vi "STAGE+mono+counter_edit20.vi"() -> ()   [LabVIEW 2017]
panel:
  out "PROGRESS":u8(slide) max=10 step=10 scale=0.0..100.0
  in  "?":enum32{"Page 1", "Page 2"}(tab)
  out "XY Graph":cluster{dbl[], dbl[]}(graph)
  out "XY Graph 2":cluster{dbl[], dbl[]}[](graph)
  in  "Collect Data!":bool
  out "Timeout":bool
  in  "?":bool
  out "Timeout 2":bool
  out "Waveform Graph":waveform(dbl)[](graph)
  in  "?":enum32{"DELAY", "COUNTER", "MONO", "PLOT"}(tab)
  out "Final time [ps]":dbl
  out "Current time [ps]":dbl
  out "Initial time [ps]":dbl
  in  "Set this as t0":bool
  in  "Axis":i32=1
  in  "Motor ON":bool
  in  "Motor OFF":bool
  out "Current Position [mm]":dbl
  out "Final Position [mm]":dbl
  in  "Data Points":i32=100
  out "Current Point":i32
  in  "Step Size [um]":i32=10
  in  "Target [mm]":dbl format="%.3f"
  in  "Move":bool
  out "Initial position [mm]":dbl
  in  "GPIB address":string="23"
  in  "Count Mode":u16(ring) items=["A,B for Preset T", "A-B for Preset T", "A+B for Preset T", "A for Preset B"]
  in  "Trigger mode":u16(ring) items=["10 MHz"=0, "Input 2"=2, "Input T"=3]
  in  "Channel A Input":u16(ring)=1 items=["10 MHz", "Input 1"]
  in  "Channel B Input":u16(ring)=2 items=["Input 1"=1, "Input 2"=2]
  in  "Number of Measurements\n to take at one point/ Number of Periods":u16=1 min=1 max=2000 step=1
  in  "Time between measurements\n at one point (s)/Dwell Time":dbl=0.002 min=0.002 max=60.0 step=0.001
  in  "gate mode (CW:0)":i16(slide) scale=0.0..2.0 scale format="%.2f"
  out "Counts":i32
  in  "Integrating time \nin 10^-7 sec":dbl=10000000.0
  in  "Discriminator Level (mV)":dbl min=-300.0 max=300.0 step=0.2
  in  "Discriminator Slope":bool
  in  "Channel":i16 min=0 max=2 step=1
  out "Grating #":dbl
  out "Blaze angle":dbl
  out "Grooves/mm":dbl
  out "Mono port":T1(ring)
  out "Time delay":u32=450000 min=1
  in  "Step size":dbl=10.0 min=0.0
  in  "Scan to":i32=4000
  in  "Scan from":i32=2600
  out "Current wavelength":dbl
  in  "?":bool
  in  "Array":dbl[](array[numeric])
  out "Numeric":i32
  out "Numeric 2":i32
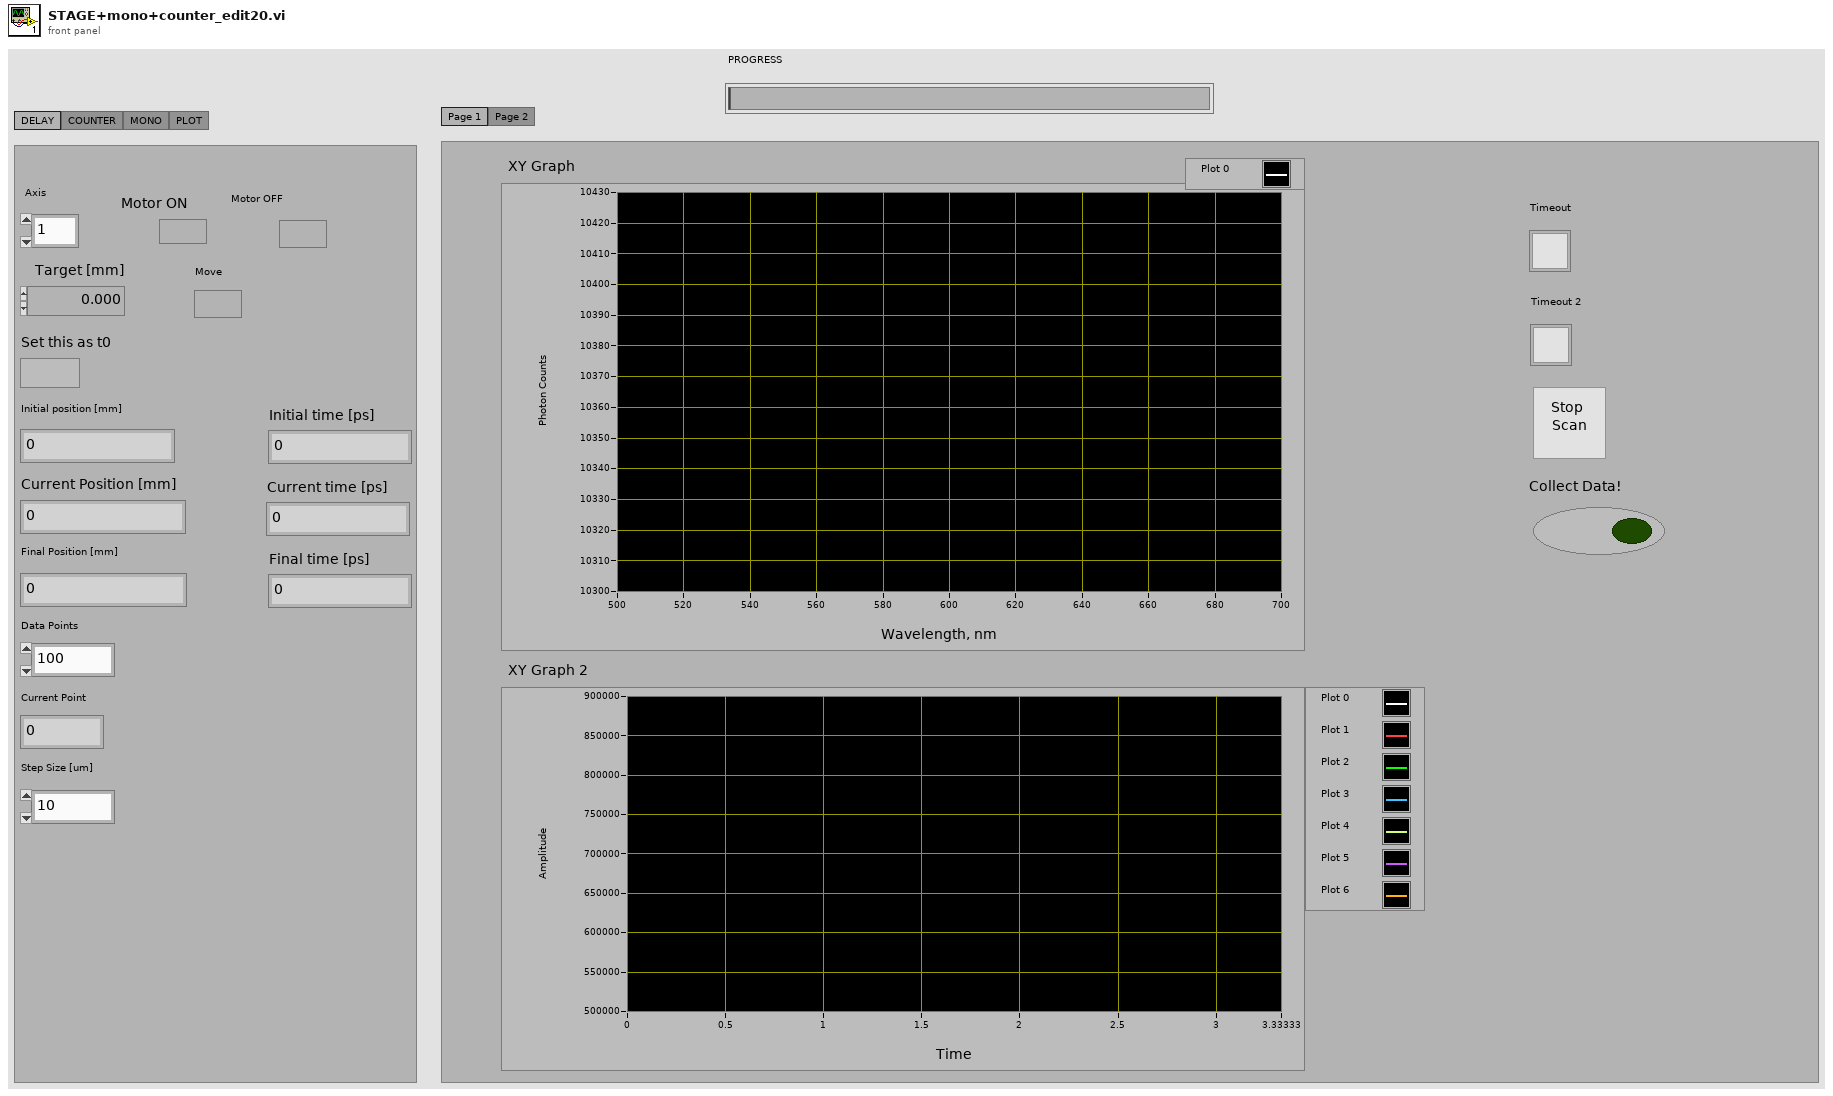
[diagram p1: front panel]
types:
  T1 = enum8{"COM 1", "COM 2", "COM 3", "COM 4", "COM 5", "COM 6", "COM 7", "COM 8", "COM 9"}
  T2 = cluster{"input XON/XOFF":bool, "input HW Handshake":bool, "input alt HW HShk":bool, "output XON/XOFF":bool, "output HW Handshake":bool, "output alt HW HShk":bool, "XOFF byte":u8, "XON byte":u8, "parity error byte":u16}
  T3 = enum16{"no parity", "odd parity", "even parity", "mark parity", "space parity"}
  T4 = typedef "NI_Matrix.lvlib/RealMatrix.ctl" = dbl[][]
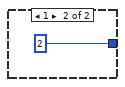
[diagram p5: hidden frame]
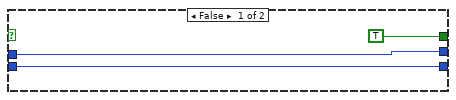
[diagram p6: hidden frame]
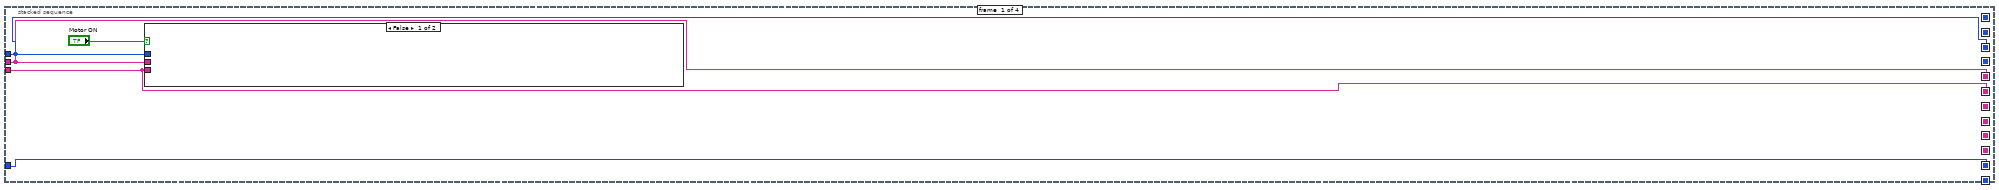
[diagram p7: hidden frame]
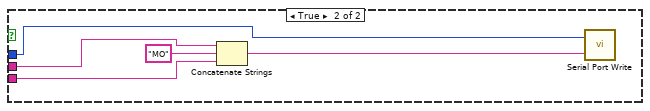
[diagram p8: hidden frame]
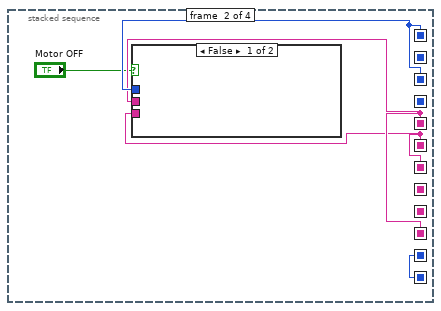
[diagram p9: hidden frame]
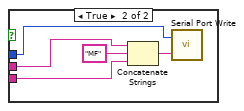
[diagram p10: hidden frame]
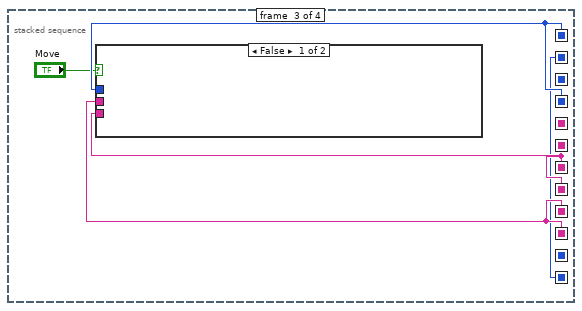
[diagram p11: hidden frame]
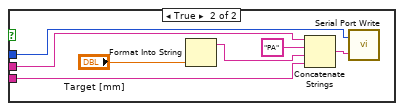
[diagram p12: hidden frame]
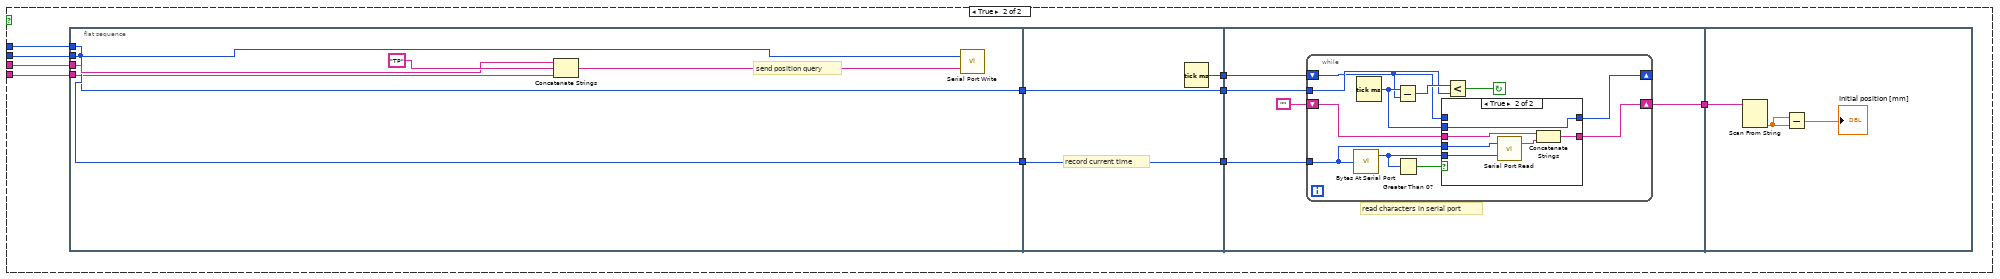
[diagram p13: hidden frame]
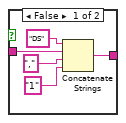
[diagram p15: hidden frame]
diagram:
  (unwired) FALSE
  w41 = u32 19200  # baud rate
  w40 = u16 8  # data bits
  w39 = enum16{"1 bit", "1.5 bits", "2 bits"}."1 bit"  # stop bits
  w43 = T3."no parity"  # parity
  w38 = 4  # 0=COM1 so n=COM(n+1)
  w42 = u16 1024  # buffer size
  n1 = flat-sequence {
    tunnel: ["Data Points"] -> w47
    tunnel: "Axis" -> [w69]
    tunnel: [w61] -> w46
    tunnel: [w69] -> w45
    tunnel: ["Step Size [um]"] -> w19
    tunnel: [w61] -> w18
    tunnel: ["Step Size [um]"] -> w17
    tunnel: ["Data Points"] -> w16
    tunnel: [w61] -> w15
    tunnel: [w60] -> w14
    tunnel: [w61] -> w12
    tunnel: [w60] -> w11
    tunnel: [w63] -> w10
    tunnel: [w52] -> w9
    tunnel: [w53] -> w2
    tunnel: [w52] -> w1
    tunnel: w47 -> [w161]
    tunnel: w46 -> [w160]
    tunnel: w45 -> [w159]
    tunnel: w38 -> [w155]
    tunnel: "GPIB address" -> [w154]
    tunnel: "GPIB address" -> [w153]
    tunnel: w19 -> [w142]
    tunnel: w18 -> [w140]
    tunnel: w17 -> [w139]
    tunnel: w16 -> [w137]
    tunnel: w15 -> [w132]
    tunnel: w14 -> [w131]
    tunnel: "Integrating time \nin 10^-7 sec" -> [w130]
    tunnel: w12 -> [w129]
    tunnel: w11 -> [w128]
    tunnel: w10 -> [w127]
    tunnel: w9 -> [w125]
    tunnel: w5 -> [w115]
    tunnel: w4 -> [w114]
    tunnel: w3 -> [w113]
    tunnel: w2 -> [w83]
    tunnel: w1 -> [w82]
    frame #0 {
      n2 = while {
        stop <- "Collect Data!" stop-if-true
        n3 = Multiply(x=1, y=1000) -> (x*y=w51:i32)
        n4 = Wait (ms)(milliseconds to wait=w51) -> ()  [unwired: 1 out]
      }
    }
    frame #1 {
      w54 = 1000000000000.0
      w59 = 1000
      w62 = 300000000
      w64 = 1000
      n5 = local read "Initial position [mm]"() -> (w61:dbl)
      n6 = Multiply(x="Step Size [um]", y="Data Points") -> (x*y=w68:i32)
      n7 = Divide(x=w68, y=w64) -> (x/y=w67:dbl)
      n8 = Divide(x="Step Size [um]", y=w64) -> (x/y=w63:dbl)
      n9 = Add(x=w61, y=w67) -> (x+y=w60:dbl)
      "Final Position [mm]" <- w60
      n10 = Divide(x=w60, y=w59) -> (x/y=w58:dbl)
      n11 = Divide(x=w61, y=w59) -> (x/y=w57:dbl)
      n12 = Divide(x=w58, y=w62) -> (x/y=w55:dbl)
      n13 = Divide(x=w57, y=w62) -> (x/y=w56:dbl)
      n14 = Multiply(x=w55, y=w54) -> (x*y=w53:dbl)
      "Final time [ps]" <- w53
      n15 = Multiply(x=w56, y=w54) -> (x*y=w52:dbl)
      "Initial time [ps]" <- w52
    }
    frame #2 {
      w74 = 1
      w95 = "\r\n"
      n16 = Increment(x=w137) -> (x+1=w138:i32)
      n17 = local read "Numeric 2"() -> (w78:i32)
      n18 = Multiply(x="Scan from", y=w74) -> (x*y=w70:i32)
      n19 = Multiply(x="Scan to", y=w74) -> (x*y=w72:i32)
      n20 = local read "Numeric"() -> (w77:i32)
      n21 = Divide(x=w142, y=1000.0) -> (x/y=w119:dbl)
      n22 = for {
        N: w138 -> [_]
        tunnel: w119 -> [w172]
        tunnel: w140 -> [w170]
        tunnel: [w163] -> w136 mode=indexing
        i -> [w171]
        # "distances"
        n23 = Multiply(x=w172, y=w171) -> (x*y=w169:dbl)
        n24 = Add(x=w170, y=w169) -> (x+y=w168:dbl)
        n25 = Divide(x=w168, y=1000) -> (x/y=w162:dbl)
        n26 = Divide(x=w162, y=300000000) -> (x/y=w165:dbl)
        n27 = Multiply(x=w165, y=1000000000000.0) -> (x*y=w163:dbl)
      }
      n28 = To Time Stamp(1:w70) -> (0:w86:timestamp)
      n29 = Initialize Array(0.0, w77, w78) -> ()  [unwired: 1 out]
      n30 = Multiply(x=w72, y=1) -> (x*y=w126:i32)
      n31 = Multiply(x=1, y=w70) -> (x*y=w118:i32)
      n32 = Divide(x=w119, y=1000.0) -> (x/y=w120:dbl)
      n33 = Subtract(x=w126, y=w118) -> (x-y=w148:i32)
      n34 = Divide(x=w120, y=300000000) -> (x/y=w122:dbl)
      n35 = Divide(x=w148, y="Step size") -> (x/y=w147:dbl)
      n36 = Bundle By Name("Y"=dbl[] [], "t0"=w86, "dt"="Step size") -> (w85:waveform(dbl))  [unwired: 1 in]
      n37 = property on="Waveform Graph" class="WFGraph (strict)"("XScale.Increment"="Step size", "XScale.Maximum"=w72, "XScale.Minimum"=w70) -> ()  [unwired: 2 in, 2 out]
      n38 = Multiply(x=w122, y=1000000000000.0) -> (x*y=w81:dbl)
      n39 = Build Array(w85) -> (w84:waveform(dbl)[])
      n40 = Round Toward -Infinity(1:w147) -> (0:w146:dbl)
      n41 = Concatenate Strings("\r", "\n") -> (w156:string)
      n42 = property on="XY Graph 2" class="XYGraph (strict)"("XScale.Increment"=w81, "XScale.Maximum"=w83, "XScale.Minimum"=w82) -> ()  [unwired: 2 in, 2 out]
      n43 = Increment(x=w146) -> (x+1=w117:dbl)
      n44 = for {
        N: w117 -> [_]
        tunnel: "Step size" -> [w177]
        tunnel: w118 -> [w175]
        tunnel: [w173] -> w116 mode=indexing
        i -> [w176]
        # "wavelengths"
        n45 = Multiply(x=w177, y=w176) -> (x*y=w174:dbl)
        n46 = Add(x=w175, y=w174) -> (x+y=w173:dbl)
      }
      n47 = for {
        N: w161 -> [w188]
        tunnel: w160 -> [w250]
        tunnel: w139 -> [w246]
        tunnel: w159 -> [w243]
        tunnel: w156 -> [w240]
        tunnel: w155 -> [w241]
        tunnel: w154 -> [w239]
        tunnel: w114 -> [w236]
        tunnel: w115 -> [w238]
        tunnel: w153 -> [w237]
        tunnel: [w198] -> w88 mode=indexing
        tunnel: w118 -> [w178]
        tunnel: "Step size" -> [w231]
        tunnel: w146 -> [w230]
        tunnel: w132 -> [_]
        tunnel: w131 -> [_]
        tunnel: w130 -> [w229]
        tunnel: w72 -> [w228]
        tunnel: w70 -> [w227]
        tunnel: "Step size" -> [w204]
        tunnel: w129 -> [w220]
        tunnel: w128 -> [w218]
        tunnel: w127 -> [w221]
        tunnel: w81 -> [w190]
        tunnel: w125 -> [w225]
        tunnel: w70 -> [w205]
        tunnel: "Step size" -> [w206]
        shift-right: [w189] -> _
        shift-left: dbl[] [] -> [w184]
        tunnel: w115 -> [w203]
        tunnel: w114 -> [w202]
        tunnel: w113 -> [w201]
        shift-right: [w195] -> _
        shift-left: w84 -> [w196]
        shift-right: [w182] -> _
        shift-left: dbl[][] [] -> [w181]
        i -> [w187]
        w200 = dbl[] []
        w219 = 1000
        w222 = 300000000
        n48 = stacked-sequence {
          tunnel: w236 -> [w471]
          tunnel: w237 -> [_]
          frame #0 {
            n49 = call <vilib>:"Close Serial Driver.vi"("port number"=w471) -> ()  [unwired: 1 out]
            n50 = GPIB Misc(0:"loc 23" ("command string")) -> ()  [unwired: 1 in, 3 out]
          }
        }
        n51 = property on="PROGRESS" class="Slide (strict)"("Scale.Increment"=1, "Scale.Maximum"=w188, "Scale.Minimum"=0) -> ()  [unwired: 2 in, 2 out]
        n52 = flat-sequence {
          tunnel: w239 -> [w276]
          tunnel: w238 -> [w275]
          tunnel: w236 -> [w274]
          tunnel: w178 -> [w273]
          tunnel: w231 -> [w272]
          tunnel: w230 -> [w271]
          tunnel: w228 -> [w270]
          tunnel: w227 -> [w269]
          tunnel: w200 -> [w268]
          tunnel: w200 -> [w267]
          tunnel: w206 -> [w266]
          tunnel: w205 -> [w265]
          tunnel: w204 -> [w264]
          tunnel: w203 -> [w263]
          tunnel: w202 -> [w262]
          tunnel: w201 -> [w261]
          tunnel: [w259] -> w199
          tunnel: [w260] -> _
          tunnel: [w259] -> w197
          tunnel: [w451] -> w198
          tunnel: w199 -> [w451]
          tunnel: [w450] -> w183
          tunnel: [w449] -> w180
          frame #0 {
            # "step size"
            n53 = while {
              tunnel: w274 -> [_]
              tunnel: w275 -> [_]
              tunnel: w276 -> [w285]
              tunnel: w273 -> [w312]
              tunnel: w272 -> [w278]
              tunnel: w271 -> [w311]
              tunnel: w270 -> [w281]
              tunnel: w269 -> [w280]
              tunnel: w264 -> [w282]
              tunnel: w266 -> [w309]
              shift-right: [w305] -> w259
              shift-left: w267 -> [w304]
              shift-right: [w299] -> w260
              shift-left: w268 -> [w307]
              tunnel: w265 -> [w302]
              tunnel: w263 -> [w289]
              tunnel: w262 -> [w288]
              tunnel: w261 -> [w287]
              i -> [w310]
              stop <- w315 stop-if-true
              n54 = property on="XY Graph" class="XYGraph (strict)"("XScale.Increment"=w282, "XScale.Maximum"=w281, "XScale.Minimum"=w280) -> ()  [unwired: 2 in, 2 out]
              n55 = Multiply(x=1, y=w278) -> (x*y=w277:dbl)
              n56 = Multiply(x=w310, y=w309) -> (x*y=w308:dbl)
              n57 = Multiply(x=w310, y=w277) -> (x*y=w316:dbl)
              n58 = Greater Or Equal?(x=w310, y=w311) -> (x >= y?=w313:bool)
              n59 = Add(x=w308, y=w302) -> ()  [unwired: 1 out]
              n60 = Add(x=w316, y=w312) -> (x+y=w286:dbl)
              n61 = Or(x="?", y=w313) -> (x .or. y?=w315:bool)
              n62 = Build Array (concatenate)(w307, w286) -> (w306:dbl[])
              n63 = flat-sequence {
                tunnel: w285 -> [w334]
                tunnel: w286 -> [w335]
                tunnel: [w335] -> w293
                tunnel: [w324] -> w292
                tunnel: [w323] -> w291
                tunnel: [w334] -> w290
                tunnel: w289 -> [w327]
                tunnel: w288 -> [w326]
                tunnel: w287 -> [w325]
                tunnel: [w374] -> w298
                tunnel: [w373] -> w297
                tunnel: [w371] -> w296
                tunnel: w293 -> [w369]
                tunnel: w292 -> [w374]
                tunnel: w291 -> [w373]
                tunnel: w290 -> [w371]
                tunnel: w298 -> [w381]
                tunnel: w297 -> [w380]
                tunnel: w296 -> [w375]
                tunnel: [w375] -> w284
                tunnel: w284 -> [w383]
                tunnel: [w383] -> w283
                tunnel: w283 -> [w436]
                tunnel: [w436] -> w295
                tunnel: w295 -> [w437]
                tunnel: [w437] -> w294
                tunnel: [w443] -> w301
                tunnel: w294 -> [w444]
                frame #0 {
                  n64 = flat-sequence {
                    tunnel: w327 -> [w341]
                    tunnel: [w341] -> w333
                    tunnel: w326 -> [w343]
                    tunnel: [w343] -> w332
                    tunnel: w325 -> [w339]
                    tunnel: [w339] -> w331
                    tunnel: w333 -> [w347]
                    tunnel: [w347] -> w322
                    tunnel: w332 -> [w348]
                    tunnel: [w348] -> w320
                    tunnel: w331 -> [w345]
                    tunnel: [w345] -> w318
                    tunnel: w322 -> [w352]
                    tunnel: [w352] -> w321
                    tunnel: w320 -> [w351]
                    tunnel: [w351] -> w319
                    tunnel: w318 -> [w350]
                    tunnel: [w350] -> w317
                    tunnel: w321 -> [w359]
                    tunnel: [w359] -> w330
                    tunnel: w319 -> [w356]
                    tunnel: [w356] -> w329
                    tunnel: w317 -> [w354]
                    tunnel: [w354] -> w328
                    tunnel: w330 -> [w361]
                    tunnel: w329 -> [w362]
                    tunnel: w328 -> [_]
                    tunnel: [w362] -> w324
                    tunnel: [w361] -> w323
                    frame #0 {
                      n65 = call "Query11x.vi"("port number"=w343, "QUERY"=u16 0, "time delay"=w341) -> ("timeout"=w340:bool, "STATUS MESSAGE"=w338:u16)  [unwired: 2 out]
                      n66 = local write "Timeout"(w340) -> ()
                      n67 = Divide(x=w338, y=10 ("Numeric")) -> (x/y=→"Current wavelength":dbl)
                    }
                    frame #1 {
                      n68 = call "Query11x.vi"("port number"=w348, "QUERY"=u16 2, "time delay"=w347) -> ("timeout"=w346:bool, "STATUS MESSAGE"=→"Grooves/mm":u16)  [unwired: 2 out]
                      n69 = local write "Timeout"(w346) -> ()
                    }
                    frame #2 {
                    }
                    frame #3 {
                      n70 = Divide(x=w359, y=i16 100 ("device (1)")) -> (x/y=w357:dbl)
                      n71 = call "Query11x.vi"("port number"=w356, "QUERY"=u16 3, "time delay"=w357) -> ("timeout"=w355:bool, "STATUS MESSAGE"=→"Blaze angle":u16)  [unwired: 2 out]
                      n72 = local write "Timeout"(w355) -> ()
                    }
                    frame #4 {
                      n73 = Divide(x=w361, y=i16 100 ("device (1)")) -> (x/y=w365:dbl)
                      n74 = call "Query11x.vi"("port number"=w362, "QUERY"=u16 4, "time delay"=w365) -> ("timeout"=w364:bool, "STATUS MESSAGE"=→"Grating #":u16)  [unwired: 2 out]
                      n75 = local write "Timeout"(w364) -> ()
                    }
                  }
                }
                frame #1 {
                  n76 = Multiply(x=w369, y=10) -> (x*y=w368:dbl)
                  n77 = call "Goto11x.vi"("time delay"=w373, "WAVELENGTH"=w368, "port number"=w374) -> ("timeout"=w372:bool)  [unwired: 2 out]
                  n78 = local write "Timeout 2"(w372) -> ()
                }
                frame #2 {
                  # "set counter time in 10^-7 seconds in CW"
                  n79 = call "Query11x.vi"("port number"=w381, "QUERY"=0, "time delay"=w380) -> ("timeout"=w379:bool, "STATUS MESSAGE"=w378:u16)  [unwired: 2 out]
                  n80 = local write "Timeout 2"(w379) -> ()
                  n81 = Divide(x=w378, y=10) -> (x/y=w377:dbl)
                  n82 = local write "Current wavelength"(w377) -> ()
                }
                frame #3 {
                  # "Configures discriminator."
                  n83 = flat-sequence {
                    tunnel: w383 -> [w393]
                    tunnel: [w393] -> w392
                    tunnel: [w400] -> w391
                    tunnel: [w398] -> w390
                    tunnel: "Discriminator Slope" -> [w399]
                    tunnel: w392 -> [w398]
                    tunnel: w384 -> [w397]
                    tunnel: w391 -> [w419]
                    tunnel: [w420] -> w389
                    tunnel: w390 -> [w418]
                    tunnel: [w418] -> w388
                    tunnel: w384 -> [w416]
                    tunnel: w389 -> [w432]
                    tunnel: w388 -> [w431]
                    tunnel: "Discriminator Level (mV)" -> [w426]
                    tunnel: w384 -> [w425]
                    frame #0 {
                      # "Flush I/O buffers."
                      n84 = for {
                        N: 5 -> [_]
                        tunnel: w393 -> [w395]
                        n85 = GPIB Write(0:w395, 1:"\r") -> ()  [unwired: 3 in, 2 out]
                      }
                    }
                    frame #1 {
                      # "Set discriminator slope."
                      n86 = case shown="True" w399 {
                        tunnel: [w406 w411] -> w401
                        tunnel: w397 -> [w405 w410]
                        frame False {
                          n87 = Concatenate Strings("DS", w405, ",", "1") -> (w406:string)
                        }
                        frame True {
                          n88 = Concatenate Strings("DS", w410, ",", "0") -> (w411:string)
                        }
                      }
                      n89 = GPIB Write(0:w398, 1:w401, 2:5) -> (6:w400:errorcluster)  [unwired: 2 in, 1 out]
                    }
                    frame #2 {
                      # "Set discriminator mode to fixed."
                      n90 = Concatenate Strings("DM", w416, ",", "0") -> (w415:string)
                      n91 = GPIB Write(0:w418, 1:w415, 2:5, 3:w419) -> (6:w420:errorcluster)  [unwired: 1 in, 1 out]
                    }
                    frame #3 {
                      # "Set discriminator level.\nMust be between +300 and -300 mV."
                      n92 = Divide(x=w426, y=1000.0) -> (x/y=w434:dbl)
                      n93 = Number To Fractional String(number=w434, precision (6)=i16 4) -> (F-format string=w423:string)  [unwired: 2 in]
                      n94 = Concatenate Strings("DL", w425, ",", w423) -> (w430:string)
                      n95 = GPIB Write(0:w431, 1:w430, 2:5, 3:w432) -> (6:w427:errorcluster)  [unwired: 1 in, 1 out]
                      n96 = call <vilib>:"General Error Handler.vi"("type of dialog (OK msg:1)"=1, "error in (no error)"=w427) -> ()  [unwired: 9 in, 5 out]
                    }
                  }
                  n97 = Number To Decimal String(number="Channel") -> (decimal integer string=w384:string)  [unwired: 1 in]
                }
                frame #4 {
                  n98 = call "Start.vi"("GPIB Address"=w436) -> ()  [unwired: 9 in]
                }
                frame #5 {
                  # "Wait for Scan to Finish"
                  n99 = for {
                    N: 1 -> [_]
                    tunnel: w437 -> [w439]
                    n100 = while {
                      tunnel: w439 -> [w440]
                      stop <- w442 stop-if-true
                      n101 = call "ScanDone.vi"("Wait (ms)"=1000, "GPIB Address"=w440) -> ("Scan Finished?"=w442:bool)
                    }
                  }
                }
                frame #6 {
                  n102 = call "Read Data.vi"("Channel Number"=0, "GPIB Address"=w444, "Number of Datapoints"=1) -> ("Data"=w445:i32[])
                  n103 = Index Array(array=w445, index=0) -> (element=w443:i32)
                  "Counts" <- w443
                }
              }
              n104 = Build Array (concatenate)(w304, w301) -> (w303:dbl[])
              n105 = Bundle(w306, w303) -> (w300:cluster{dbl[], dbl[]})  [unwired: 1 in]
              "XY Graph" <- w300
              n106 = Unbundle(w300) -> (w299:dbl[], w305:dbl[])
            }
          }
          frame #1 {
            n107 = Array Size(array="Array") -> (size(s)=w449:i32)
            n108 = flat-sequence {
              tunnel: w451 -> [w457]
              tunnel: "Array" -> [w456]
              tunnel: w449 -> [w455]
              tunnel: [w453] -> w450
              frame #0 {
                n109 = for {
                  N: w455 -> [w462]
                  tunnel: w456 -> [w469]
                  tunnel: w457 -> [w464]
                  shift-right: [w458] -> w453
                  shift-left: dbl[] [] -> [w459]
                  i -> [w461]
                  n110 = local read "Scan from"() -> (w467:i32)
                  n111 = Index Array(array=w469, index=w461) -> (element=w468:dbl)
                  n112 = local read "Step size"() -> (w465:dbl)
                  n113 = Subtract(x=w468, y=w467) -> (x-y=w466:dbl)
                  n114 = Divide(x=w466, y=w465) -> (x/y=w463:dbl)
                  n115 = Index Array(array=w464, index=w463) -> (element=w460:dbl)
                  n116 = Insert Into Array(array=w459, index=w461, new element=w460) -> (w458:dbl[])
                  "Numeric" <- w462
                }
              }
            }
          }
        }
        n117 = Divide(x=w220, y=w219) -> (x/y=w216:dbl)
        n118 = Divide(x=w218, y=w219) -> (x/y=w215:dbl)
        n119 = Divide(x=w221, y=w219) -> (x/y=w217:dbl)
        n120 = Multiply(x=w190, y=w187) -> (x*y=w226:dbl)
        n121 = Number To Decimal String(number=w229) -> (decimal integer string=w234:string)  [unwired: 1 in]
        n122 = Add(x=1, y=w187) -> (x+y=→"PROGRESS":i32)
        n123 = Divide(x=w246, y=1000) -> (x/y=w245:dbl)
        n124 = Divide(x=w216, y=w222) -> (x/y=w210:dbl)
        n125 = Divide(x=w215, y=w222) -> (x/y=w209:dbl)
        n126 = Divide(x=w217, y=w222) -> (x/y=w211:dbl)
        n127 = Add(x=w225, y=w226) -> (x+y=w185:dbl)
        n128 = Concatenate Strings("CP 2,", w234) -> (w232:string)
        n129 = Multiply(x=w210, y=1000000000000.0) -> ()  [unwired: 1 out]
        n130 = Multiply(x=w209, y=1000000000000.0) -> ()  [unwired: 1 out]
        n131 = Multiply(x=w211, y=1000000000000.0) -> ()  [unwired: 1 out]
        n132 = Multiply(x=w245, y=w187) -> (x*y=w249:dbl)
        n133 = Build Array (concatenate)(w184, w185) -> (w186:dbl[])
        n134 = Add(x=w250, y=w249) -> (x+y=w248:dbl)
        n135 = Format Into String(w243) -> (resulting string=w242:string)  [unwired: 3 in, 1 out]
        n136 = GPIB Write(0:w239, 1:w232, 2:i16 5 ("mode (0)")) -> ()  [unwired: 2 in, 2 out]
        n137 = flat-sequence {
          tunnel: w248 -> [w474]
          tunnel: [w474] -> w244
          tunnel: w240 -> [w476]
          tunnel: w242 -> [w475]
          tunnel: w241 -> [w472]
          tunnel: w244 -> [w485]
          frame #0 {
            n138 = Format Into String(w474) -> (resulting string=w473:string)  [unwired: 3 in, 1 out]
            n139 = Wait (ms)(milliseconds to wait=u32 100) -> ()  [unwired: 1 out]
            n140 = Concatenate Strings(w475, "PA" ("Substring"), w473, w476) -> (w478:string)
            n141 = call <vilib>:"Serial Port Write.vi"("string to write"=w478, "port number"=w472) -> ()  [unwired: 1 out]
          }
          frame #1 {
            n142 = Divide(x=w485, y=1000) -> (x/y=w483:dbl)
            n143 = Wait (ms)(milliseconds to wait=u32 1000) -> ()  [unwired: 1 out]
            n144 = Divide(x=w483, y=300000000) -> (x/y=w482:dbl)
            n145 = Multiply(x=w482, y=1000000000000.0) -> (x*y=→"Current time [ps]":dbl)
            "Current Position [mm]" <- w485
          }
        }
        n146 = local read "Scan from"() -> (w193:i32)
        n147 = local read "Step size"() -> (w191:dbl)
        n148 = To Time Stamp(1:w193) -> (0:w192:timestamp)
        n149 = Bundle By Name("Y"=w197, "t0"=w192, "dt"=w191) -> (w194:waveform(dbl))  [unwired: 1 in]
        n150 = Build Array (concatenate)(w196, w194) -> (w195:waveform(dbl)[])
        "Waveform Graph" <- w195
        n151 = for {
          N: w180 -> [_]
          tunnel: [w258] -> w189
          tunnel: w186 -> [w257]
          tunnel: w183 -> [w255]
          tunnel: [w254] -> w182
          tunnel: w181 -> [w256]
          tunnel: [w251] -> w179 mode=indexing
          i -> [w253]
          n152 = Build Array (concatenate)(w256, w255) -> (w254:dbl[][])
          n153 = Index Array(array=w255, index=w253) -> ()  [unwired: 1 out]
          n154 = Index Array(array=w254, index (col)=w253) -> (element=w252:dbl[])  [unwired: 1 in]
          n155 = Bundle(w257, w252) -> (w251:cluster{dbl[], dbl[]})  [unwired: 1 in]
          n156 = Unbundle(w251) -> (w258:dbl[])  [unwired: 1 out]
        }
        "XY Graph 2" <- w179
        "Current Point" <- w187
        "Numeric 2" <- w188
      }
      n157 = Build Array (concatenate)(0, w136) -> (w89:dbl[])
      n158 = local read "Integrating time \nin 10^-7 sec"() -> (w93:dbl)
      n159 = Build Array(w116) -> (w145:dbl[][])
      n160 = Transpose Matrix(1:w145) -> (0:w144:dbl[][])
      n161 = Transpose Matrix(1:w88) -> (0:w143:dbl[][])
      n162 = Build Array (concatenate)(w144, w143) -> (w90:T4)
      n163 = Insert Into Array(array=w90, index (row)=0, new element=w89) -> (w133:T4)  [unwired: 1 in]
      n164 = local read "Blaze angle"() -> (w112:dbl)
      n165 = local read "Grating #"() -> (w111:dbl)
      n166 = Multiply(x=w93, y=1e-07) -> (x*y=w92:dbl)
      n167 = Get Date/Time In Seconds() -> (seconds since 1Jan1904=w105:timestamp)
      n168 = Array To Spreadsheet String(delimiter (Tab)=",", array=w133, 3:"%f" ("format string")) -> (spreadsheet string=w94:string)
      n169 = Format Date/Time String(time format string (%c)="%Y-%b-%d %H:%M:%S", seconds (now)=w105) -> (date/time string=w106:string)  [unwired: 1 in]
      n170 = Number To Decimal String(number=w92) -> (decimal integer string=w107:string)  [unwired: 1 in]
      n171 = Number To Decimal String(number=w111) -> (decimal integer string=w108:string)  [unwired: 1 in]
      n172 = Number To Decimal String(number=w112) -> (decimal integer string=w96:string)  [unwired: 1 in]
      n173 = call <vilib>:"Space Constant.vi"() -> ("String"=w109:string)
      n174 = Concatenate Strings(w95, "Data was taken on ", w106, w95, "Integration Time is ", w107, w109, "s", w95, "Monochromator gratng # ", w108, "; ", "blazed for ", w96, w109, "nm", w95, w95, w95, w94) -> (w110:string)
      n175 = Write to Text File(text=w110) -> ()  [unwired: 3 in, 3 out]
    }
  }
  n176 = flat-sequence {
    tunnel: [w489] -> w32
    tunnel: [w488] -> w31
    frame #0 {
      n177 = call "CM Com Read ini.vi"() -> ("Mono port"=w488:T1, "time delay1"=w489:u32)  [unwired: 7 in]
    }
  }
  n178 = call <vilib>:"Serial Port Init.vi"("flow control etc."=T2 {"input XON/XOFF"=FALSE, "input HW Handshake"=FALSE, "input alt HW HShk"=FALSE, "output XON/XOFF"=FALSE, "output HW Handshake"=FALSE, "output alt HW HShk"=FALSE, "XOFF byte"=13, "XON byte"=11, "parity error byte"=0}, "parity"=w43, "buffer size"=w42, "stop bits"=w39, "data bits"=w40, "baud rate"=w41, "port number"=w38) -> ("error code"=w37:i32)
  n179 = call "CM Serial Port Setup.vi"("COM port"=w31, "time delay"=w32) -> ("time delay1"=w27:u32, "DK port Out"=w28:T1, "error code"=w30:i32)  [unwired: 7 in]
  n180 = Equal To 0?(x=w30) -> (x = 0?=w29:bool)
  n181 = Concatenate Strings("\r", "\n") -> (w33:string)
  n182 = while {
    tunnel: w38 -> [w492]
    tunnel: w33 -> [w493]
    tunnel: w37 -> [_]
    tunnel: "Axis" -> [w490]
    stop <- TRUE continue-if-true
    w491 = u32 200  # timeout
    n183 = Format Into String(w490) -> (resulting string=w494:string)  [unwired: 3 in, 1 out]
    n184 = stacked-sequence {
      seq-local: [w499 _ _ _] -> [_ w510 _ _]
      seq-local: [w498 _ _ _] -> [_ w509 _ _]
      seq-local: [w500 _ _ _] -> [_ w511 _ _]
      seq-local: [w497 _ _ _] -> [_ w507 _ _]
      seq-local: [_ w510 _ _] -> [_ _ w520 _]
      seq-local: [_ w509 _ _] -> [_ _ w519 _]
      seq-local: [_ w511 _ _] -> [_ _ w521 _]
      seq-local: [_ w507 _ _] -> [_ _ w517 _]
      seq-local: [_ _ w520 _] -> [_ _ _ w533]
      seq-local: [_ _ w519 _] -> [_ _ _ w530]
      seq-local: [_ _ w521 _] -> [_ _ _ w532]
      seq-local: [_ _ w517 _] -> [_ _ _ w531]
      tunnel: w494 -> [w499 _ _ _]
      tunnel: w493 -> [w498 _ _ _]
      tunnel: w492 -> [w500 _ _ _]
      tunnel: w491 -> [w497 _ _ _]
      frame #0 {
        n185 = case shown="False" "Motor ON" {
          tunnel: w500 -> [_ w506]
          tunnel: w499 -> [_ w503]
          tunnel: w498 -> [_ w502]
          frame False {
          }
          frame True {
            n186 = Concatenate Strings(w503, "MO" ("Substring"), w502) -> (w504:string)
            n187 = call <vilib>:"Serial Port Write.vi"("string to write"=w504, "port number"=w506) -> ()  [unwired: 1 out]
          }
        }
      }
      frame #1 {
        n188 = case shown="False" "Motor OFF" {
          tunnel: w511 -> [_ w516]
          tunnel: w510 -> [_ w513]
          tunnel: w509 -> [_ w512]
          frame False {
          }
          frame True {
            n189 = Concatenate Strings(w513, "MF" ("Substring"), w512) -> (w514:string)
            n190 = call <vilib>:"Serial Port Write.vi"("string to write"=w514, "port number"=w516) -> ()  [unwired: 1 out]
          }
        }
      }
      frame #2 {
        n191 = case shown="False" "Move" {
          tunnel: w521 -> [_ w528]
          tunnel: w520 -> [_ w525]
          tunnel: w519 -> [_ w524]
          frame False {
          }
          frame True {
            n192 = Format Into String("Target [mm]") -> (resulting string=w522:string)  [unwired: 3 in, 1 out]
            n193 = Concatenate Strings(w525, "PA" ("Substring"), w522, w524) -> (w526:string)
            n194 = call <vilib>:"Serial Port Write.vi"("string to write"=w526, "port number"=w528) -> ()  [unwired: 1 out]
          }
        }
      }
      frame #3 {
        n195 = case shown="False" "Set this as t0" {
          tunnel: w533 -> [_ w543]
          tunnel: w532 -> [_ w542]
          tunnel: w531 -> [_ w541]
          tunnel: w530 -> [_ w540]
          frame False {
          }
          frame True {
            n196 = flat-sequence {
              tunnel: w543 -> [w547]
              tunnel: w542 -> [w546]
              tunnel: [w546] -> w539
              tunnel: w541 -> [w544]
              tunnel: [w544] -> w538
              tunnel: w540 -> [w545]
              tunnel: w539 -> [w551]
              tunnel: [w551] -> w537
              tunnel: w538 -> [w550]
              tunnel: [w550] -> w536
              tunnel: [w552] -> w535
              tunnel: w537 -> [w557]
              tunnel: w536 -> [w555]
              tunnel: w535 -> [w554]
              tunnel: [w553] -> w534
              tunnel: w534 -> [w579]
              frame #0 {
                # "send position query"
                n197 = Concatenate Strings(w547, "TP" ("Substring"), w545) -> (w548:string)
                n198 = call <vilib>:"Serial Port Write.vi"("string to write"=w548, "port number"=w546) -> ()  [unwired: 1 out]
              }
              frame #1 {
                # "record current time"
                n199 = Tick Count (ms)() -> (millisecond timer value=w552:u32)
              }
              frame #2 {
                # "read characters in serial port"
                n200 = while {
                  shift-left: w554 -> [w558]
                  shift-right: [w559] -> _
                  tunnel: w555 -> [w562]
                  shift-left: "" -> [w565]
                  shift-right: [w564] -> w553
                  tunnel: w557 -> [w566]
                  stop <- w561 continue-if-true
                  n201 = call <vilib>:"Bytes At Serial Port.vi"("port number"=w566) -> ("byte count"=w567:u32)  [unwired: 1 out]
                  n202 = Tick Count (ms)() -> (millisecond timer value=w560:u32)
                  n203 = Subtract(x=w560, y=w558) -> (x-y=w563:u32)
                  n204 = Greater Than 0?(x=w567) -> (x > 0?=w568:bool)
                  n205 = case shown="True" w568 {
                    tunnel: w567 -> [_ w576]
                    tunnel: w566 -> [_ w575]
                    tunnel: w565 -> [w570 w573]
                    tunnel: [w570 w572] -> w564
                    tunnel: [w569 w571] -> w559
                    tunnel: w560 -> [_ w571]
                    tunnel: w558 -> [w569 _]
                    frame False {
                    }
                    frame True {
                      n206 = call <vilib>:"Serial Port Read.vi"("requested byte count"=w576, "port number"=w575) -> ("string read"=w574:string)  [unwired: 1 out]
                      n207 = Concatenate Strings(w573, w574) -> (w572:string)
                    }
                  }
                  n208 = Less?(x=w563, y=w562) -> (x < y?=w561:bool)
                }
              }
              frame #3 {
                n209 = Scan From String(input string=w579) -> (output 1=w577:dbl)  [unwired: 4 in, 3 out]
                n210 = Subtract(x=w577, y=w577) -> (x-y=→"Initial position [mm]":dbl)
              }
            }
          }
        }
      }
    }
    n211 = Wait Until Next ms Multiple(millisecond multiple=u32 50) -> ()  [unwired: 1 out]
  }
  n212 = case shown="True" w29 {
    tunnel: w28 -> [w582 w585]
    tunnel: w27 -> [w581 w584]
    tunnel: [w582 w585] -> w4
    tunnel: [w581 w584] -> w5
    tunnel: [TRUE FALSE] -> w3
    frame False {
    }
    frame True {
      n213 = call "CM Com Write ini.vi"("time delay1"=w585, "Mono port"=w584) -> ()  [unwired: 7 in]
      n214 = local write "Mono port"(w585) -> ()
      n215 = local write "Time delay"(w584) -> ()
    }
  }
  n216 = case shown="True" "?" {
    tunnel: w5 -> [_ w587]
    tunnel: w4 -> [_ w586]
    frame False {
    }
    frame True {
      n217 = Two Button Dialog(message="Do you want to change grating?", 1:"No" ("F button name (\"Cancel\")"), 2:"Yes" ("T button name (\"OK\")")) -> (T button?=w588:bool)
      n218 = case shown="True" w588 {
        tunnel: w587 -> [_ w593]
        tunnel: w586 -> [_ w592]
        frame False {
        }
        frame True {
          n219 = Two Button Dialog(message="Disable voltage from PMT", 1:"Do not swich grating" ("F button name (\"Cancel\")"), 2:"Done" ("T button name (\"OK\")")) -> (T button?=w594:bool)
          n220 = case shown="True" w594 {
            tunnel: w593 -> [_ w615]
            tunnel: w592 -> [_ w614]
            frame False {
            }
            frame True {
              n221 = flat-sequence {
                tunnel: w615 -> [w619]
                tunnel: [w619] -> w612
                tunnel: w614 -> [w618]
                tunnel: [w618] -> w611
                tunnel: [w616] -> w610
                tunnel: w612 -> [w623]
                tunnel: [w623] -> w609
                tunnel: w611 -> [w624]
                tunnel: [w624] -> w608
                tunnel: w610 -> [w622]
                tunnel: [w622] -> w607
                tunnel: w609 -> [w630]
                tunnel: [w630] -> w603
                tunnel: w608 -> [w629]
                tunnel: [w629] -> w601
                tunnel: w607 -> [w627]
                tunnel: [w627] -> w599
                tunnel: w603 -> [w631]
                tunnel: [w631] -> w602
                tunnel: w601 -> [w632]
                tunnel: [w632] -> w600
                tunnel: w599 -> [w633]
                tunnel: [w633] -> w598
                tunnel: w602 -> [w636]
                tunnel: [w636] -> w606
                tunnel: w600 -> [w637]
                tunnel: [w637] -> w605
                tunnel: w598 -> [w635]
                tunnel: [w635] -> w604
                tunnel: w606 -> [w641]
                tunnel: w605 -> [w642]
                tunnel: [w640] -> w613
                tunnel: w604 -> [w640]
                frame #0 {
                  n222 = local read "Grating #"() -> (w617:dbl)
                  n223 = case shown="2, Default" w617 {
                    tunnel: [1 2] -> w616
                    frame 2, Default {
                    }
                    frame 1 {
                    }
                  }
                  n224 = call "Select11x2.vi"("time delay"=w619, "NEW GRT?"=w616, "port number"=w618) -> ()  [unwired: 3 out]
                }
                frame #1 {
                  n225 = call "Goto11x.vi"("time delay"=w623, "WAVELENGTH"=u16 300, "port number"=w624) -> ()  [unwired: 3 out]
                }
                frame #2 {
                  n226 = call "Query11x.vi"("port number"=w629, "QUERY"=u16 0, "time delay"=w630) -> ("STATUS MESSAGE"=w626:u16)  [unwired: 3 out]
                  n227 = local write "Current wavelength"(w626) -> ()
                }
                frame #3 {
                }
                frame #4 {
                  n228 = call "Query11x.vi"("port number"=w637, "QUERY"=u16 2, "time delay"=w636) -> ("STATUS MESSAGE"=w634:u16)  [unwired: 3 out]
                  n229 = local write "Grooves/mm"(w634) -> ()
                }
                frame #5 {
                  n230 = Divide(x=w641, y=i16 100 ("device (1)")) -> (x/y=w643:dbl)
                  n231 = call "Query11x.vi"("port number"=w642, "QUERY"=u16 3, "time delay"=w643) -> ("STATUS MESSAGE"=w639:u16)  [unwired: 3 out]
                  n232 = local write "Blaze angle"(w639) -> ()
                }
              }
              n233 = local write "Grating #"(w613) -> ()
            }
          }
        }
      }
    }
  }
  n234 = call "Configure.vi"("Dwell Time (s)"="Time between measurements\n at one point (s)/Dwell Time", "Channel T Input"="Trigger mode", "Channel B Input"="Channel B Input", "Channel A Input"="Channel A Input", "Integrating time, 10^-7 sec"="Integrating time \nin 10^-7 sec", "gate mode (CW:0)"="gate mode (CW:0)", "Scan End Mode"=FALSE, "Number of Periods"="Number of Measurements\n to take at one point/ Number of Periods", "Count Mode"="Count Mode", "GPIB Address"="GPIB address") -> ()
  "Mono port" <- w31
  "Time delay" <- w32
